vi "CountStringOccurrences.vi"(10 "Column Index":i32, 11 "Array in":string[][](array[string])) -> (3 "String Occurences out":map{string, i32}(c390))   [LabVIEW 2025]
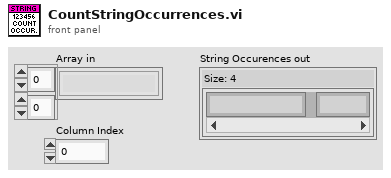
[diagram p1: front panel]
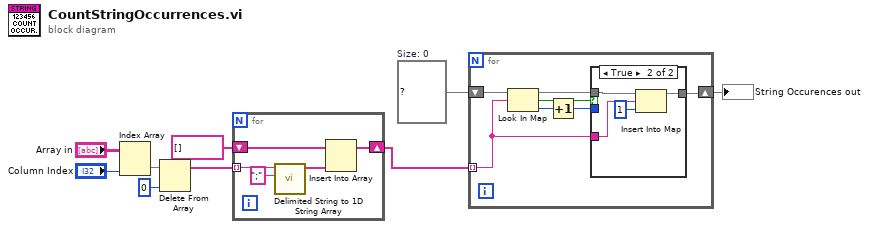
[diagram p0: block diagram]
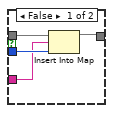
[diagram p2: hidden frame]
diagram:
  w8 = map{string, i32} {}  # Size: 0
  n1 = Index Array(array="Array in", index (col)="Column Index") -> (element=w5:string[])  [unwired: 1 in]
  n2 = Delete From Array(array=w5, index=0) -> (array with subset deleted=w3:string[])  [unwired: 1 in, 1 out]
  n3 = for {
    tunnel: w3 -> [w14] mode=indexing
    shift-right: [w10] -> w1
    shift-left: string[] [] ("string array") -> [w12]
    n4 = call <vilib>:"Delimited String to 1D String Array.vi"("delimiter"=";", "delimited string"=w14) -> ("string array"=w11:string[])  [unwired: 9 in]
    n5 = Insert Into Array(array=w12, new element=w11) -> (w10:string[])  [unwired: 1 in]
  }
  n6 = for {
    tunnel: w1 -> [w15] mode=indexing
    shift-right: [w18] -> w9
    shift-left: w8 -> [w19]
    n7 = Look In Map(map=w19, key=w15) -> (key not found?=w20:bool, value=w17:i32)  [unwired: 1 in]
    n8 = Increment(x=w17) -> (x+1=w16:i32)
    n9 = case shown="True" w20 {
      tunnel: w19 -> [w24 w28]
      tunnel: [w23 w26] -> w18
      tunnel: w16 -> [w22 _]
      tunnel: w15 -> [w21 w25]
      frame False {
        n10 = Insert Into Map(map in=w24, key=w21, value=w22) -> (map out=w23:map{string, i32})  [unwired: 2 out]
      }
      frame True {
        n11 = Insert Into Map(map in=w28, key=w25, value=1) -> (map out=w26:map{string, i32})  [unwired: 2 out]
      }
    }
  }
  "String Occurences out" <- w9
